vi "ABB Report Effy & Pass-Fail.vi"(10 "Report in":string) -> (2 "Report out":string)   [LabVIEW 2017]
uses:
  ABB global.vi
panel:
  out "Array 2":string[](array[string])
  out "Array":string[][](array[string])
  out "Selected Entries":string[][](array[string])
  out "offset past replacement":i32
  out "Efficiency Readings 2":dbl[][](array[numeric]) format="%#_4g"
  out "Efficiency Readings":dbl[][](array[numeric]) format="%#_4g"
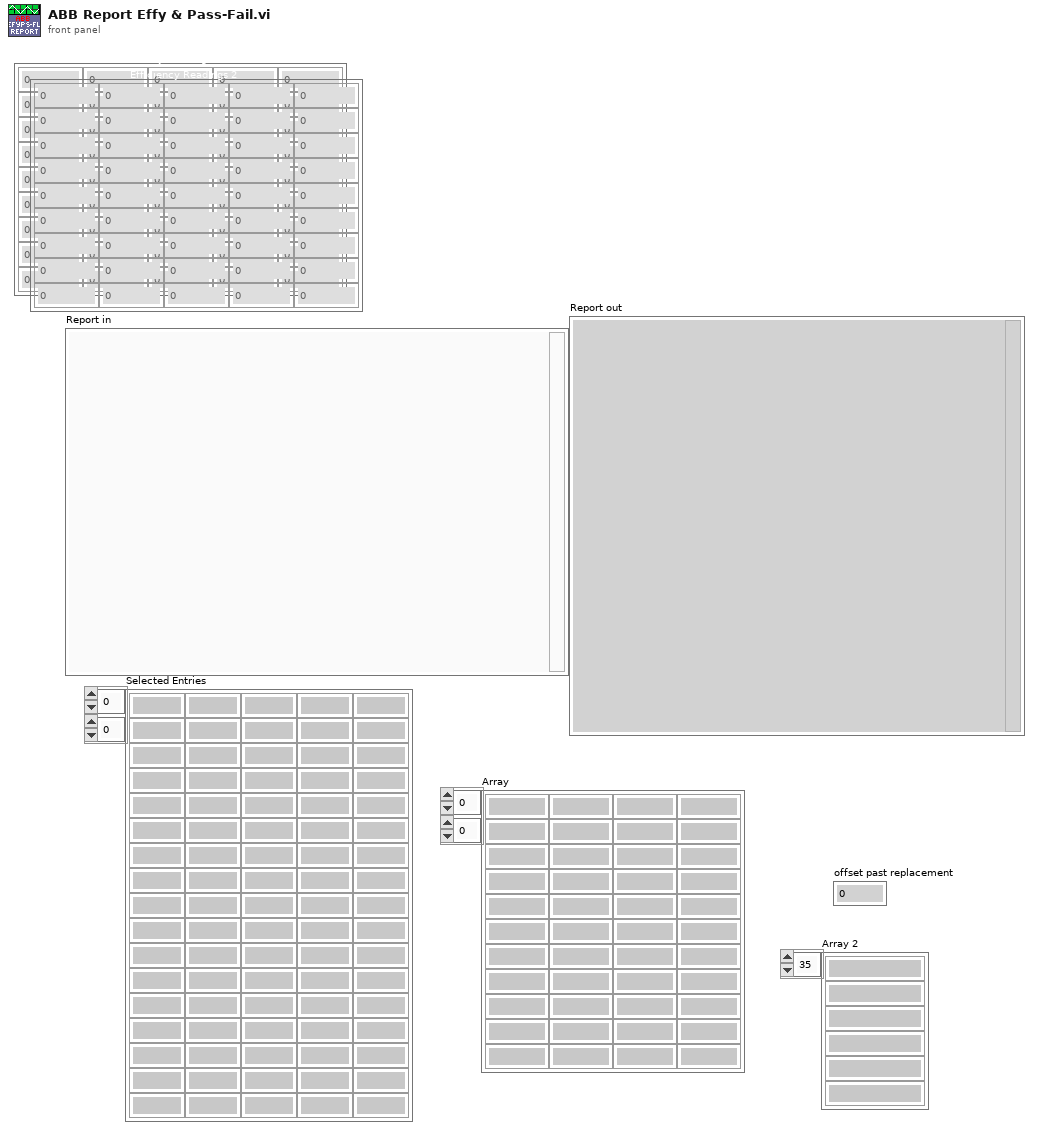
[diagram p1: front panel]
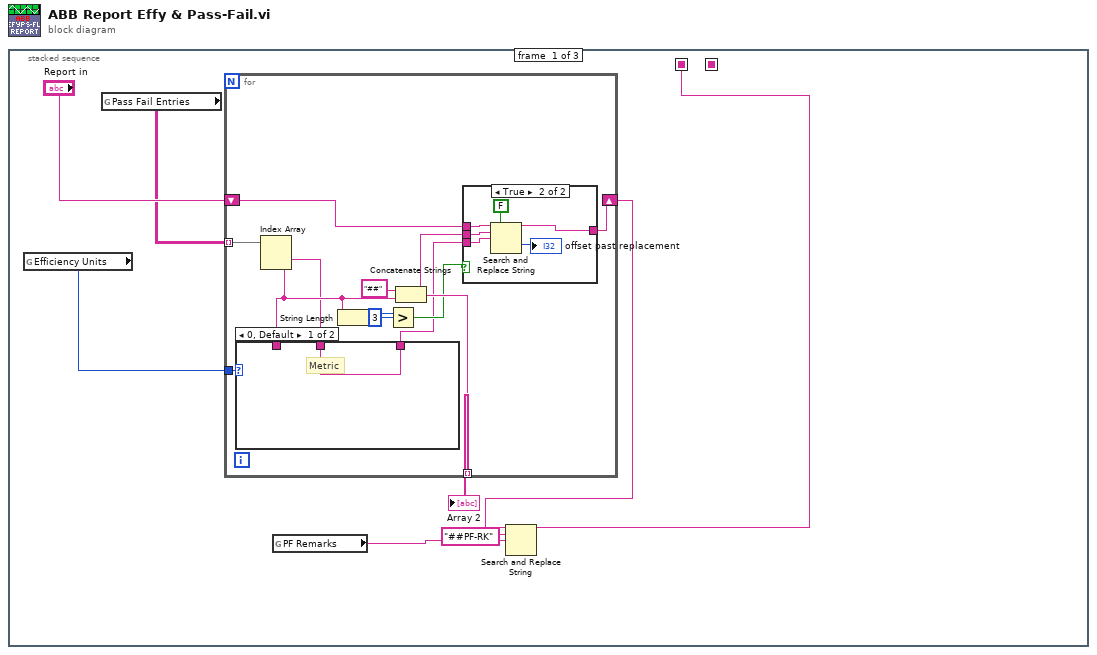
[diagram p0: block diagram]
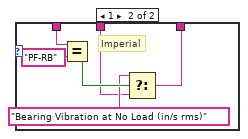
[diagram p2: hidden frame]
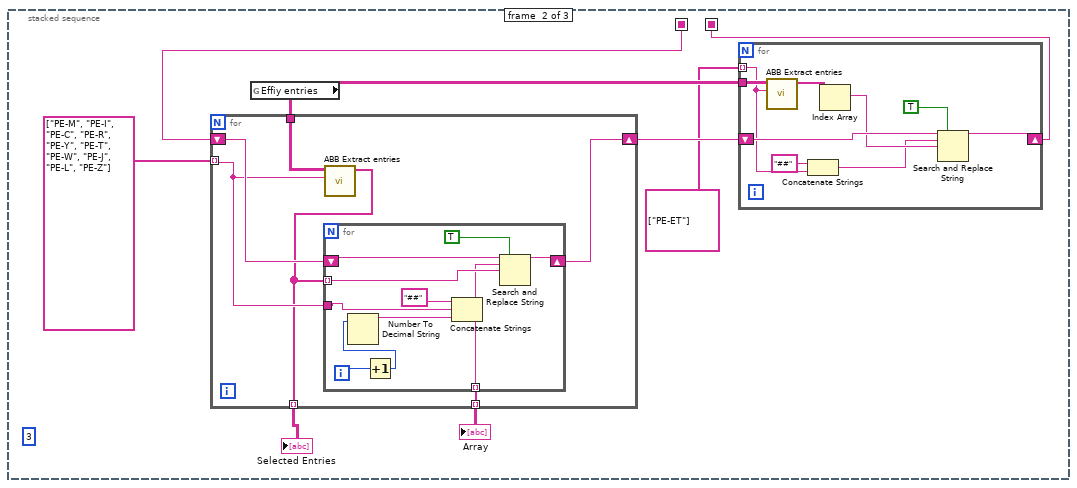
[diagram p4: hidden frame]
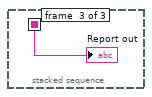
[diagram p5: hidden frame]
diagram:
  n1 = stacked-sequence {
    seq-local: [w6 _ _] -> [_ w41 _]
    seq-local: [_ w37 _] -> [_ _ w68]
    frame #0 {
      (unwired) string[] ["PE-S", "PE-M", "PE-I", "PE-C", "PE-R", "PE-Y", "PE-T", "PE-W", "PE-N"]
      (unwired) string[] ["PE-F", "PE-P", "PE-E"]
      n2 = global read "ABB global.vi" "Efficiency Units"() -> (w1:u16)
      n3 = global read "ABB global.vi" "Pass Fail Entries"() -> (w7:string[][])
      n4 = for {
        tunnel: w7 -> [w20] mode=indexing
        shift-right: [w17] -> w5
        shift-left: "Report in" -> [w18]
        tunnel: [w16] -> w2 mode=indexing
        tunnel: w1 -> [w12]
        n5 = Index Array(array=w20) -> (element #1=w10:string, element #2=w11:string)  [unwired: 2 in]
        n6 = case shown="0, Default" w12 {
          tunnel: w11 -> [_ w25]
          tunnel: [w21 w23] -> w9
          tunnel: w10 -> [w21 w22]
          frame 0, Default {
            # "Metric"
          }
          frame 1 {
            # "Imperial"
            n7 = Equal?(x=w25, y="PF-RB") -> (x = y?=w26:bool)
            n8 = Select(t="Bearing Vibration at No Load (in/s rms)", s=w26, f=w22) -> (s? t:f=w23:string)
          }
        }
        n9 = String Length(string=w11) -> (length=w15:i32)
        n10 = Greater?(x=w15, y=3) -> (0:w13:bool)
        n11 = Concatenate Strings("##" ("string"), w11) -> (w16:string)
        n12 = case shown="True" w13 {
          tunnel: w9 -> [_ w34]
          tunnel: w18 -> [w28 w33]
          tunnel: [w28 w32] -> w17
          tunnel: w16 -> [_ w29]
          frame False {
          }
          frame True {
            n13 = Search and Replace String(replace all?=FALSE ("replace all? (F)"), input string=w33, search string=w29, replace string=w34) -> (result string=w32:string, offset past replacement=→"offset past replacement":i32)  [unwired: 4 in, 2 out]
          }
        }
      }
      "Array 2" <- w2
      n14 = global read "ABB global.vi" "PF Remarks"() -> (w3:string)
      n15 = Search and Replace String(input string=w5, search string="##PF-RK", replace string=w3) -> (result string=w6:string)  [unwired: 5 in, 3 out]
    }
    frame #1 {
      (unwired) string[] ["PE-S", "PE-M", "PE-I", "PE-C", "PE-R", "PE-Y", "PE-T", "PE-W", "PE-N"]
      (unwired) string[] ["PE-F", "PE-P", "PE-E"]
      (unwired) 3 ("index")
      n16 = global read "ABB global.vi" "Effiy entries"() -> (w36:string[][])
      n17 = for {
        tunnel: string[] ["PE-M", "PE-I", "PE-C", "PE-R", "PE-Y", "PE-T", "PE-W", "PE-J", "PE-L", "PE-Z"] -> [w55] mode=indexing
        shift-right: [w54] -> w38
        shift-left: w41 -> [w56]
        tunnel: w36 -> [w57]
        tunnel: [w53] -> w40 mode=indexing
        tunnel: [w52] -> w39 mode=indexing
        n18 = call "ABB Extract entries.vi"("Entry ID"=w55, "Entry table in"=w57) -> ("Selected Entries"=w53:string[])  [unwired: 9 in]
        n19 = for {
          shift-right: [w65] -> w54
          shift-left: w56 -> [w66]
          tunnel: w53 -> [w59] mode=indexing
          tunnel: w55 -> [w63]
          tunnel: [w58] -> w52 mode=indexing
          i -> [w67]
          n20 = Increment(x=w67) -> (x+1=w61:i32)
          n21 = Number To Decimal String(number=w61) -> (decimal integer string=w60:string)  [unwired: 1 in]
          n22 = Concatenate Strings("##", w63, w60) -> (w58:string)
          n23 = Search and Replace String(replace all?=TRUE ("replace all? (F)"), input string=w66, search string=w58, replace string=w59) -> (result string=w65:string)  [unwired: 4 in, 3 out]
        }
      }
      "Selected Entries" <- w40
      "Array" <- w39
      n24 = for {
        tunnel: w36 -> [w49]
        tunnel: string[] ["PE-ET"] -> [w46] mode=indexing
        shift-right: [w50] -> w37
        shift-left: w38 -> [w51]
        n25 = call "ABB Extract entries.vi"("Entry ID"=w46, "Entry table in"=w49) -> ("Selected Entries"=w48:string[])  [unwired: 9 in]
        n26 = Concatenate Strings("##" ("string"), w46) -> (w44:string)
        n27 = Index Array(array=w48) -> (element=w47:string)  [unwired: 1 in]
        n28 = Search and Replace String(replace all?=TRUE ("replace all? (F)"), input string=w51, search string=w44, replace string=w47) -> (result string=w50:string)  [unwired: 4 in, 3 out]
      }
    }
    frame #2 {
      "Report out" <- w68
    }
  }
